vi "Single Command (2D string).vi"(8 "error in (no error)":errorcluster, 9 "Variant (Cluster, Array,..)":variant, 10 "SQL (Single Command)":string, 11 "PQ Connection in":refnum<class "PQ Connection.lvclass">) -> (0 "error out":errorcluster, 1 "Strings":string[][](array[string]), 3 "PQ Connection out":refnum<class "PQ Connection.lvclass">)   [LabVIEW 2015, in "PQ Connection.lvclass"]
uses:
  PQ Connection.lvclass
  Result/PQ Result.lvclass
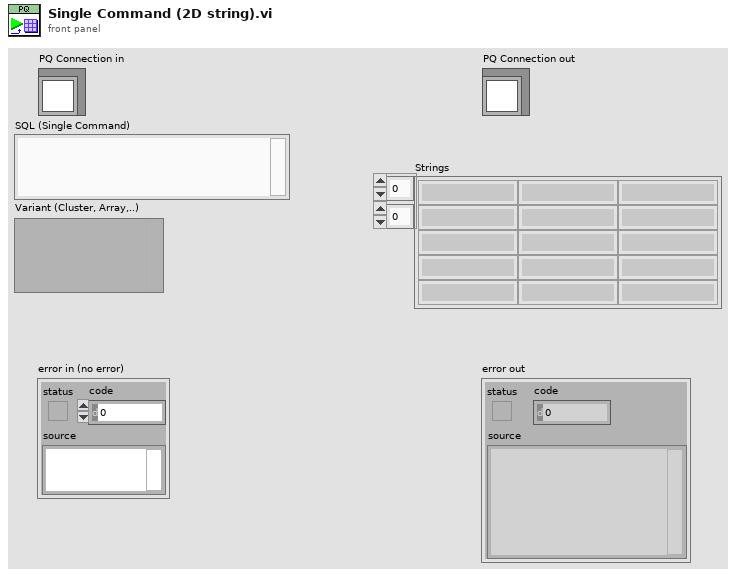
[diagram p1: front panel]
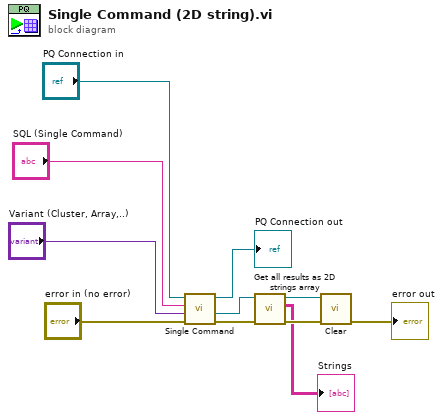
[diagram p0: block diagram]
diagram:
  n1 = call "Single Command.vi"("error in (no error)"="error in (no error)", "Variant (Cluster, Array,..)"="Variant (Cluster, Array,..)", "SQL (Single Command)"="SQL (Single Command)", "PQ Connection in"="PQ Connection in") -> ("error out"=w5:errorcluster, "First Result with Rows returned"=w4:refnum<class "PQ Result.lvclass">, "PQ Connection out"=→"PQ Connection out":refnum<class "PQ Connection.lvclass">)  [unwired: 4 in, 1 out]
  n2 = call "Get all results as 2D strings array.vi"("error in (no error)"=w5, "PQ Result in"=w4) -> ("error out"=w2:errorcluster, "Strings"=→"Strings":string[][], "PQ Result out"=w3:refnum<class "PQ Result.lvclass">)  [unwired: 7 in]
  n3 = call "Clear.vi"("error in (no error)"=w2, "PQ Result  in"=w3) -> ("error out"=→"error out":errorcluster)  [unwired: 9 in]
